vi "E5081A.vi"(5 "Input":T1={"setSweepPoint"=11, "Meas"=1, "Mark"=1, "Mark_Freq_GHz"=39.0, "Start_Freq(GHz)"=0.0, "Stop_Freq(GHz)"=0.0, "sParameter"=1}, 7 "Function_VNA":T2, 8 "error in":errorcluster, 10 "FileName":string="SENS1:CORR:CACHe:MODE 1", 11 "VISA IN":refnum<visa-resource-name>="TCPIP0::192.168.100.12::inst0::INSTR") -> (0 "error out":errorcluster, 3 "queryMarker":cluster{"gain":dbl, "phase":dbl} {"phase" format="%#.3f"; "gain" format="%#.3f"})   [LabVIEW 2023, in "Keysight.lvlib"]
uses:
  Keysight.lvlib
  CTL/Keysight_VNA.ctl
panel:
  out "Response":string
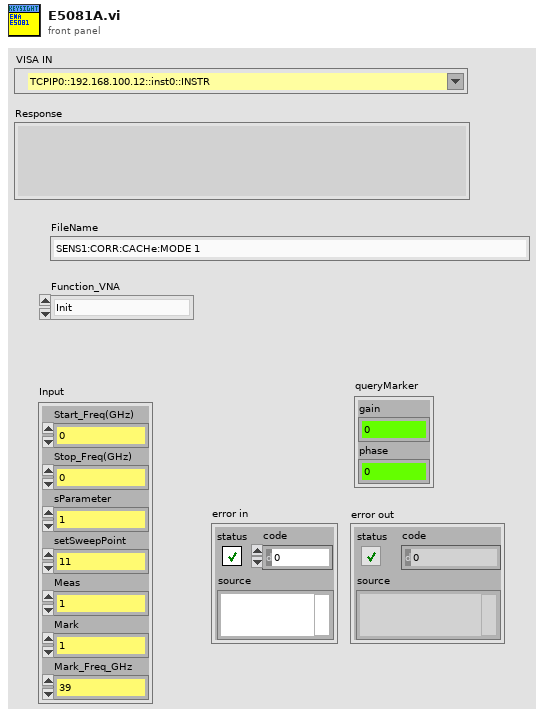
[diagram p1: front panel]
types:
  T1 = cluster{"setSweepPoint":i32, "Meas":i32, "Mark":i32, "Mark_Freq_GHz":dbl, "Start_Freq(GHz)":dbl, "Stop_Freq(GHz)":dbl, "sParameter":i32}
  T2 = typedef "Keysight_VNA.ctl" = enum16{"Init", "queryMarker", "setSweepPoint", "setMarkerFreq", "setMeasureFormat", "setFreqStartStop", "setMarkerOnOFF", "setMarkerFormat_LOGP", "setMeasPAR_S", "setTriggerSingle", "Trigger_Save_SnP", "Trigger_Single", "Close"}
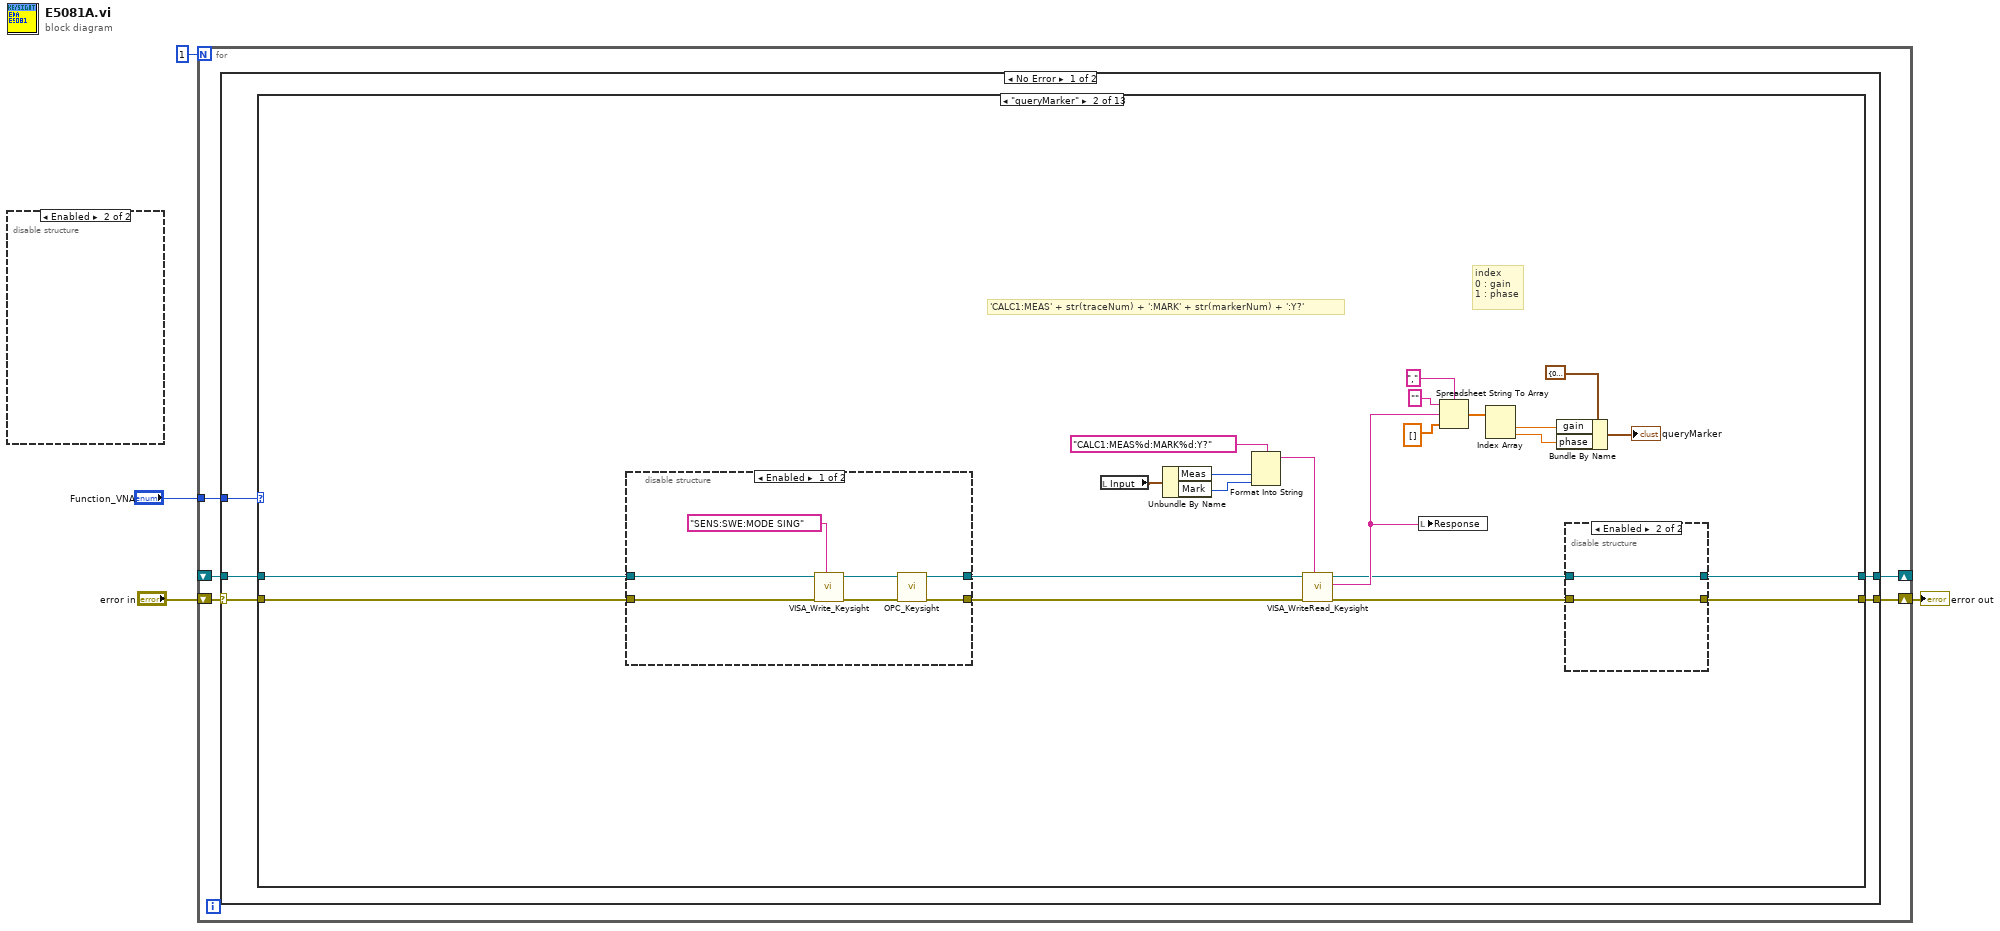
[diagram p0: block diagram]
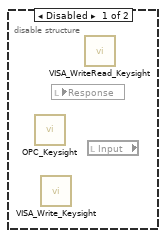
[diagram p2: hidden frame]
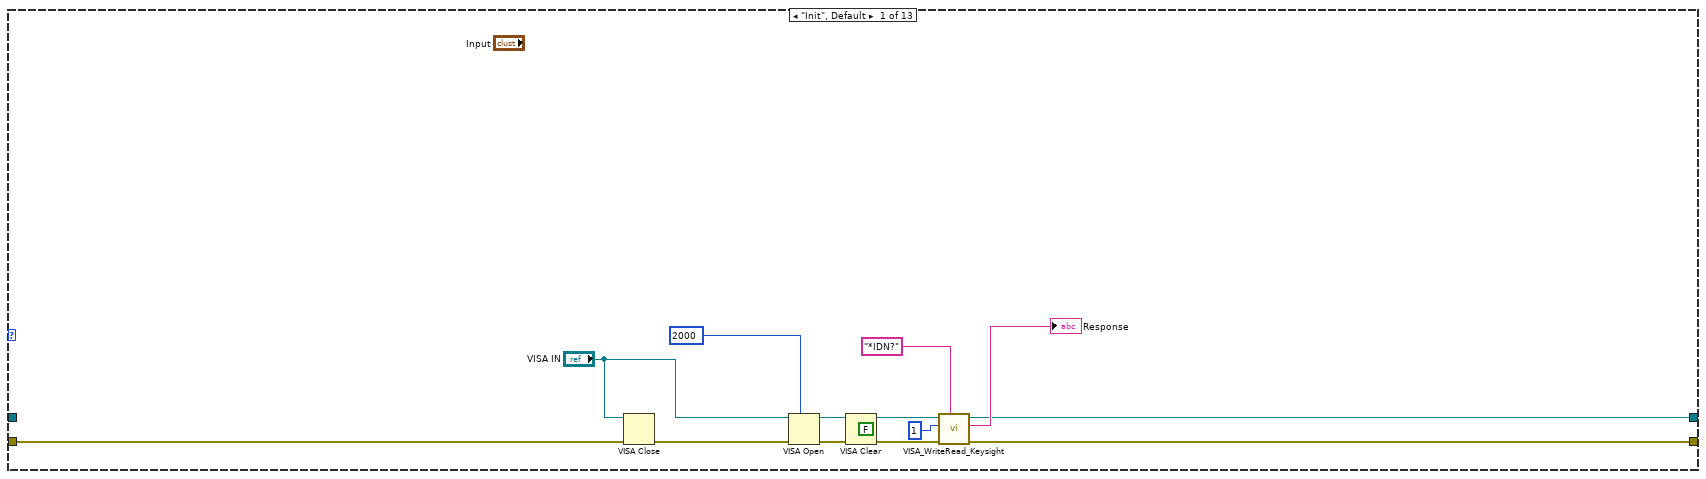
[diagram p3: hidden frame]
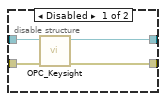
[diagram p4: hidden frame]
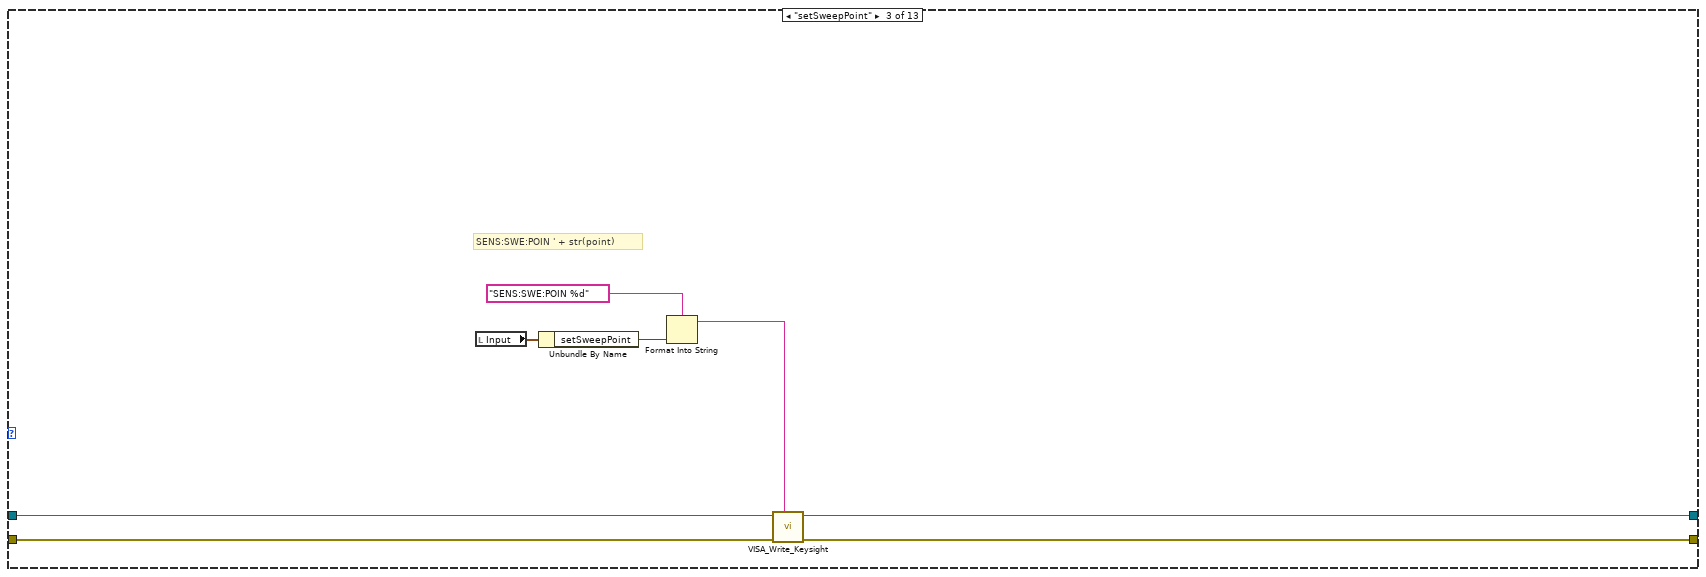
[diagram p6: hidden frame]
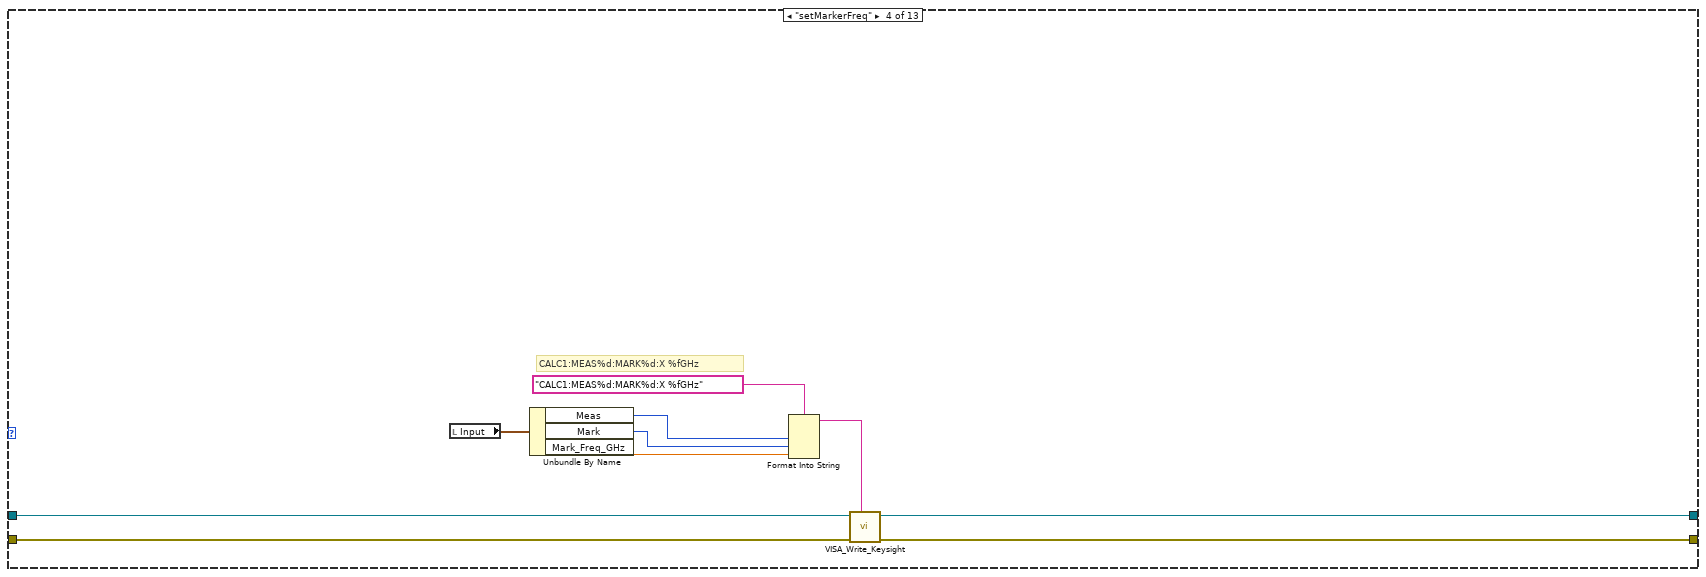
[diagram p7: hidden frame]
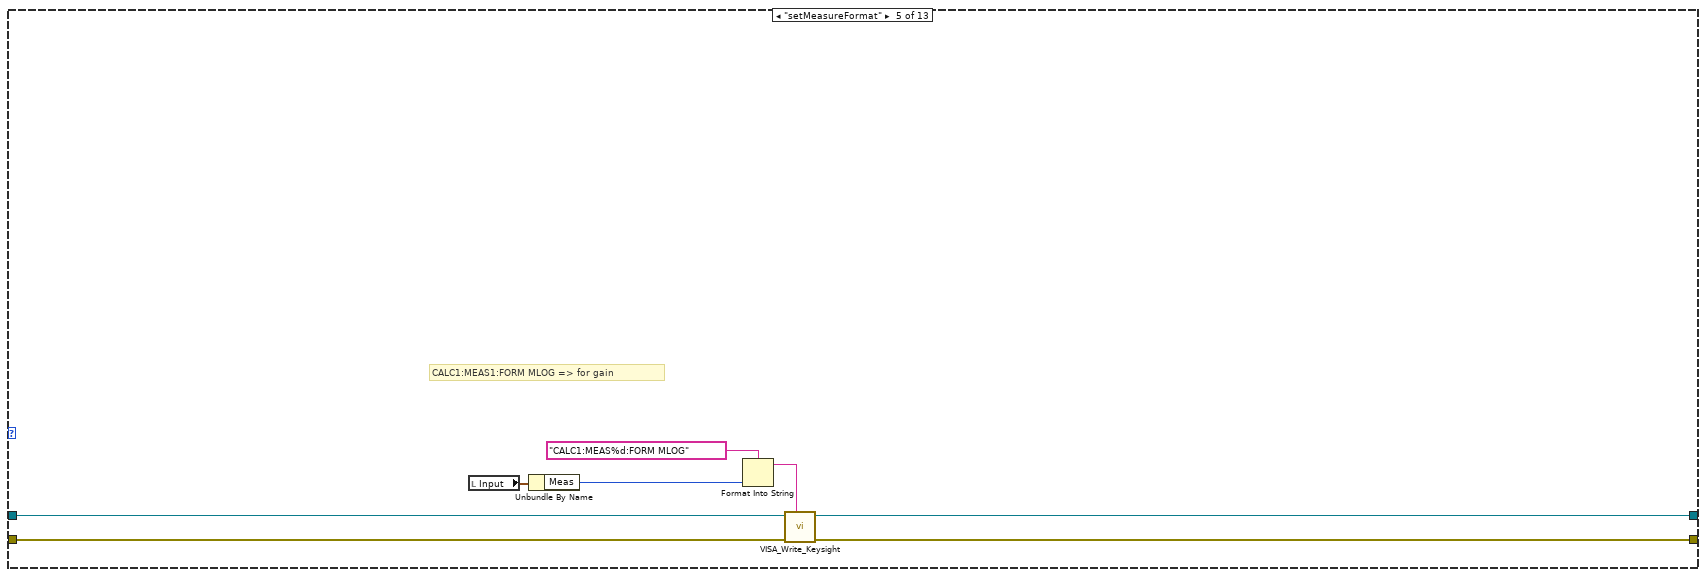
[diagram p8: hidden frame]
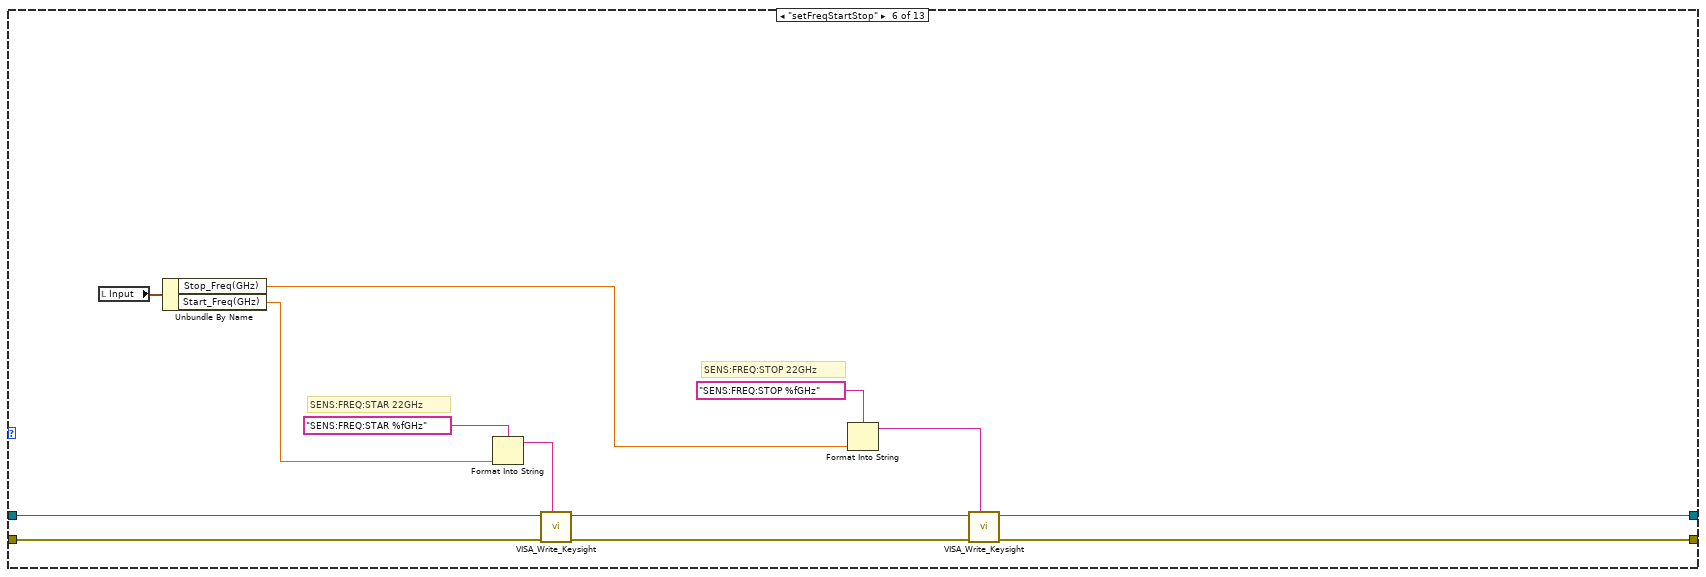
[diagram p9: hidden frame]
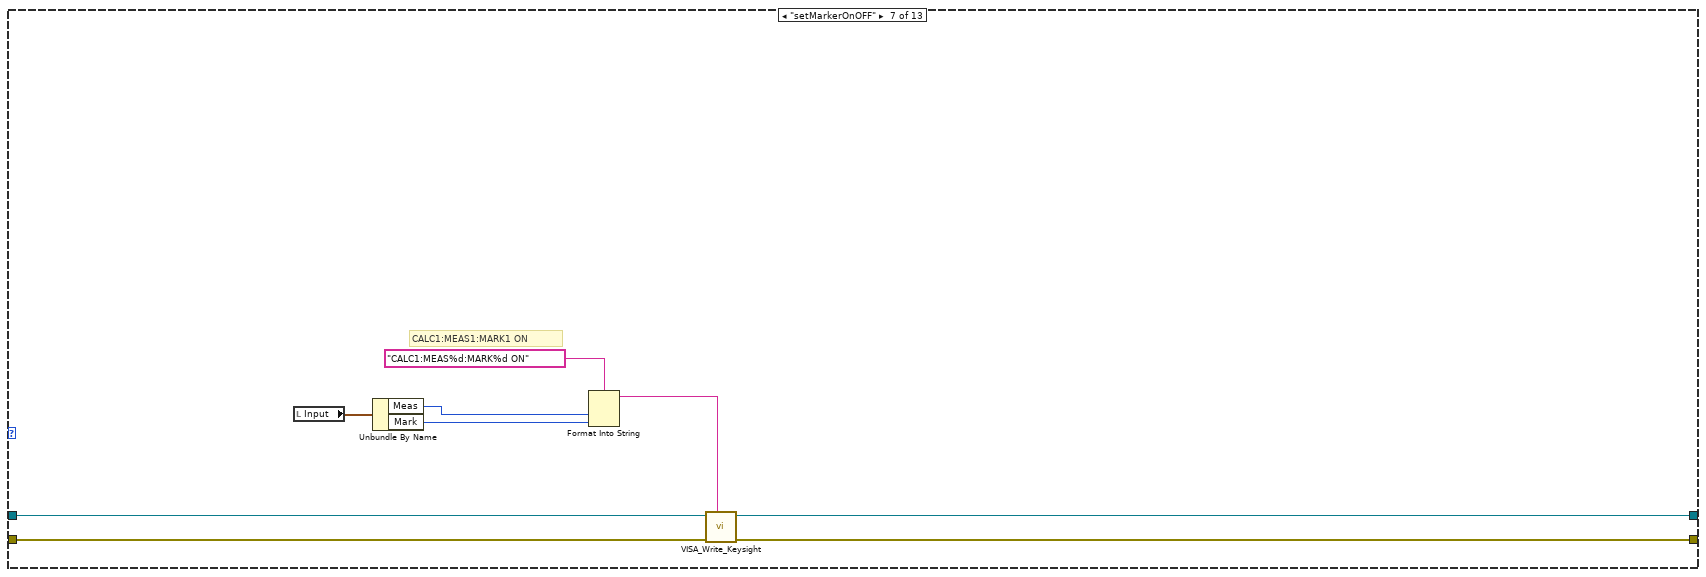
[diagram p10: hidden frame]
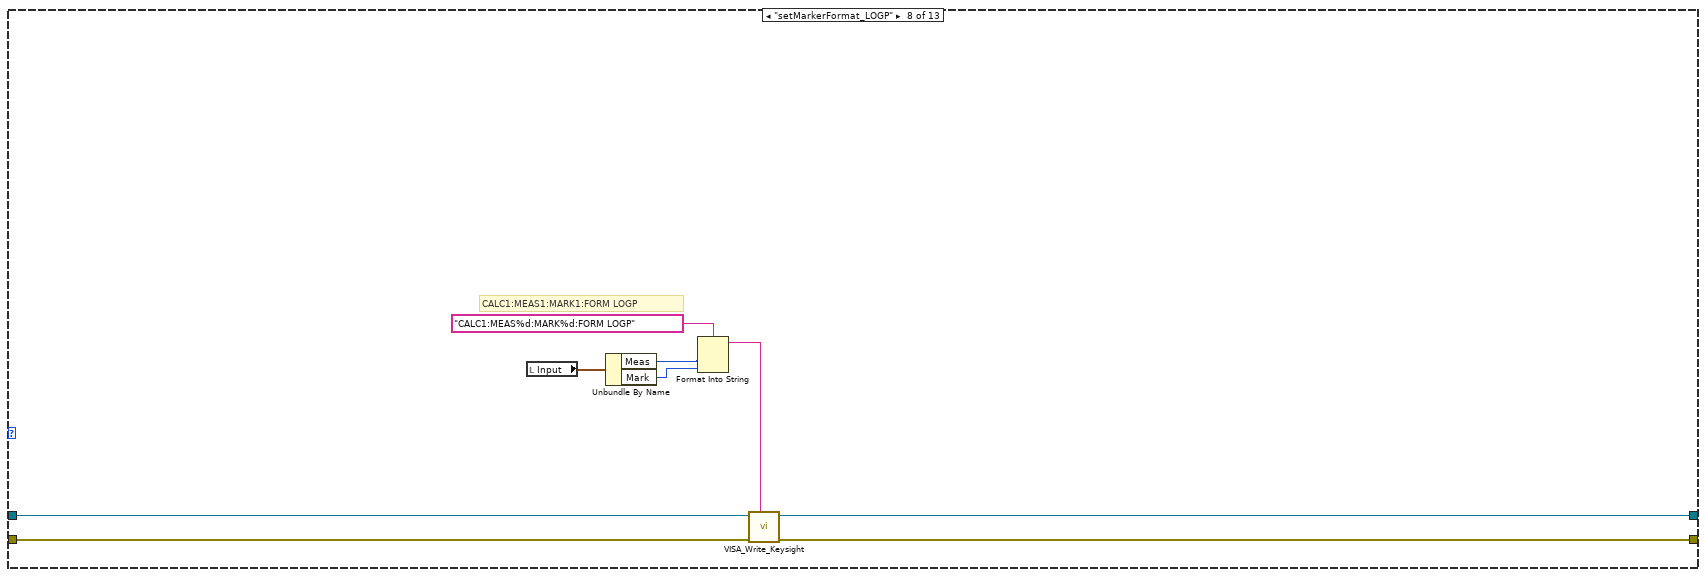
[diagram p11: hidden frame]
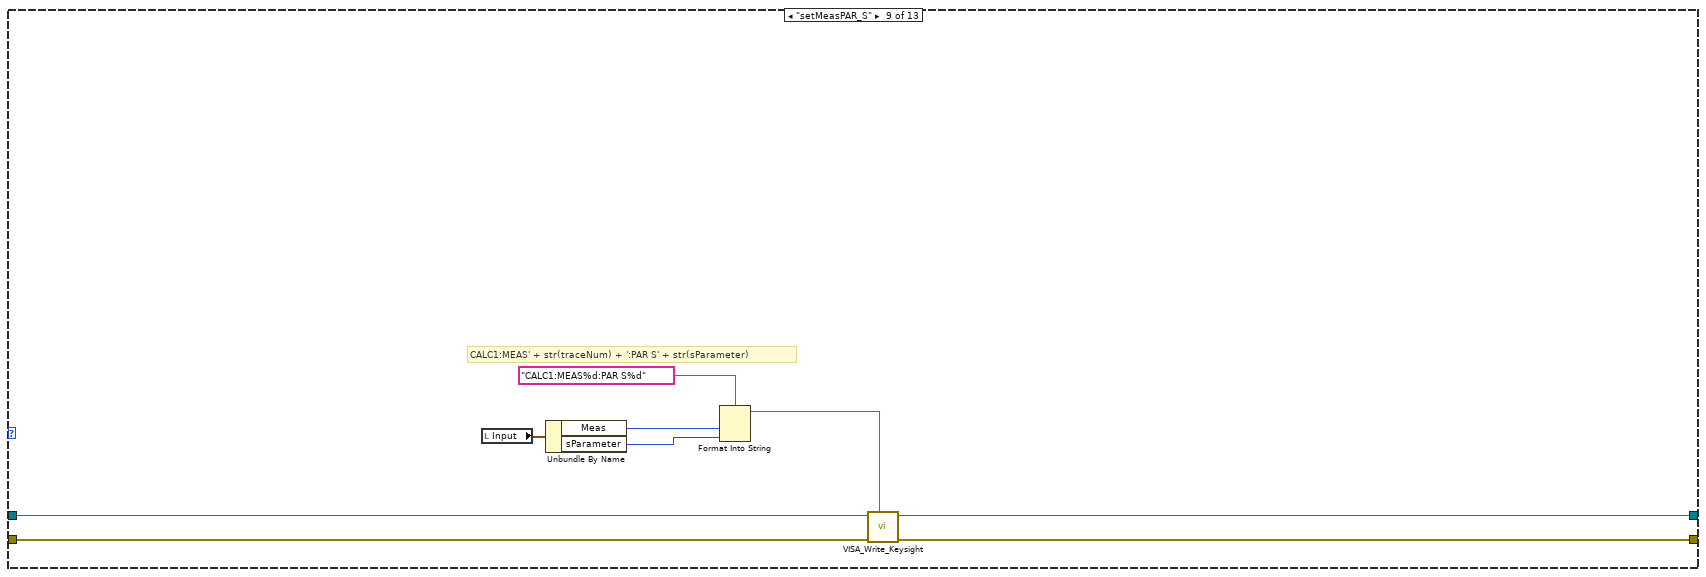
[diagram p12: hidden frame]
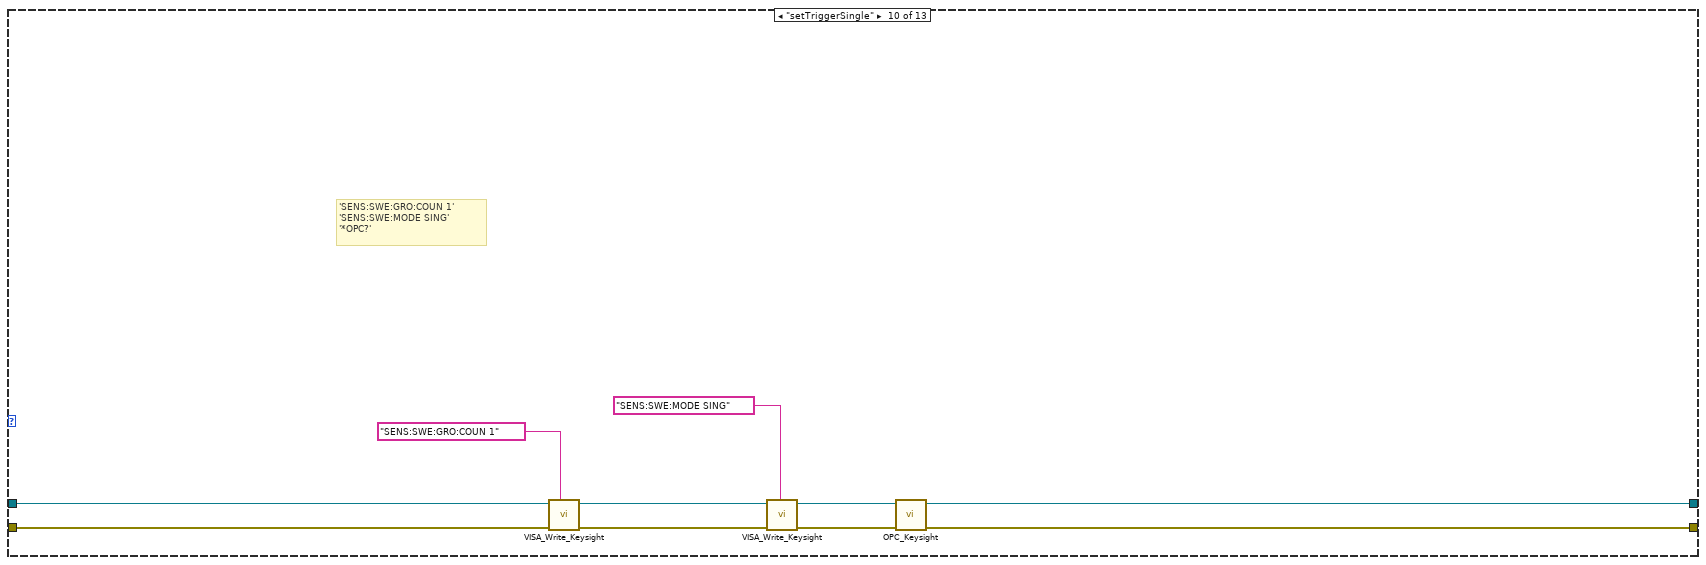
[diagram p13: hidden frame]
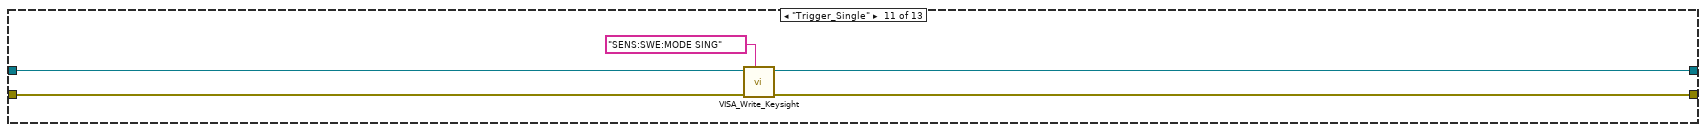
[diagram p14: hidden frame]
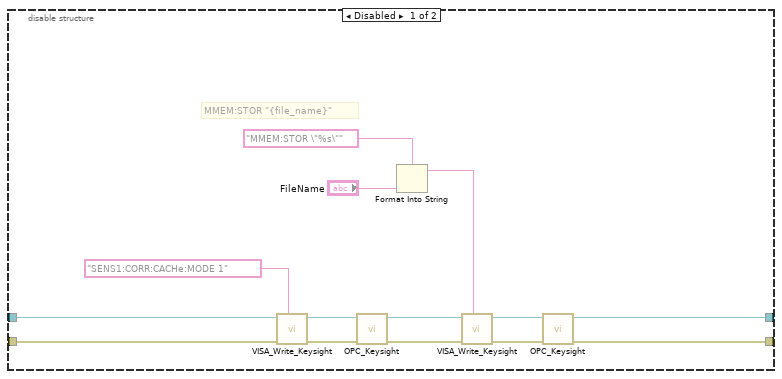
[diagram p16: hidden frame]
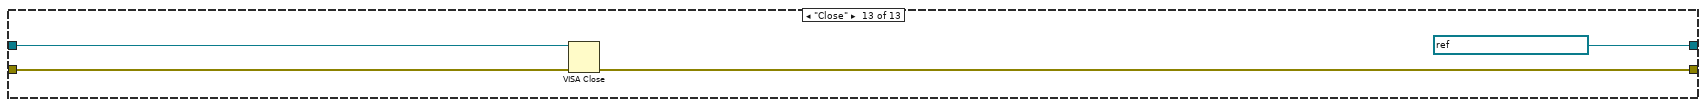
[diagram p17: hidden frame]
diagram:
  n1 = disable-structure shown="Enabled" {
    frame Disabled {
      n2 = call "OPC_Keysight.vi"() -> ()  [unwired: 10 in, 2 out]
      n3 = call "VISA_Write_Keysight.vi"() -> ()  [unwired: 10 in, 2 out]
      n4 = local read "Response"() -> ()  [unwired: 1 in]
      n5 = call "VISA_WriteRead_Keysight.vi"() -> ()  [unwired: 9 in, 3 out]
      n6 = local read "Input"() -> ()  [unwired: 1 out]
    }
    frame Enabled {
    }
  }
  n7 = for {
    N: 1 -> [_]
    tunnel: "Function_VNA" -> [w7]
    shift-right: [w8] -> w3
    shift-left: "error in" -> [w9]
    shift-right: [w5] -> _
    shift-left: _ -> [w6]
    n8 = case shown="No Error" w9 {
      selector: w9 -> [w13 w171]
      tunnel: [w11 w171] -> w8
      tunnel: w7 -> [w14 _]
      tunnel: w6 -> [w10 w170]
      tunnel: [w12 w170] -> w5
      frame No Error {
        n9 = case shown="\"queryMarker\"" w14 {
          tunnel: w13 -> [w17 w37 w70 w81 w90 w103 w112 w121 w129 w140 w144 w149 w169]
          tunnel: [w16 w34 w68 w79 w87 w95 w107 w118 w126 w134 w141 w146 refnum<visa-resource-name> refnum ("VISA out")] -> w12
          tunnel: [w15 w33 w67 w78 w89 w97 w111 w120 w128 w133 w143 w147 w167] -> w11
          tunnel: w10 -> [_ w38 w69 w80 w88 w102 w108 w119 w127 w139 w142 w148 w168]
          frame "Init", Default {
            (unwired) FALSE ("duplicate session (F)")
            n10 = VISA Close(VISA resource name="VISA IN", error in (no error)=w17) -> (error out=w24:errorcluster)
            n11 = VISA Open(timeout (0)=u32 2000 ("VISA Open timeout (0)"), error in (no error)=w24, VISA resource name="VISA IN") -> (VISA resource name=w25:refnum<visa-resource-name>, error out=w26:errorcluster)  [unwired: 2 in]
            n12 = VISA Clear(VISA resource name=w25, error in (no error)=w26) -> (VISA resource name out=w21:refnum<visa-resource-name>, error out=w22:errorcluster)
            n13 = call "VISA_WriteRead_Keysight.vi"("VISA_CMD"="*IDN?", "error in"=w22, "waiting(ms)"=u32 1, "VISA in"=w21) -> ("error out"=w15:errorcluster, "Response"=→"Response":string, "VISA out"=w16:refnum<visa-resource-name>)  [unwired: 5 in]
          }
          frame "queryMarker" {
            # "index\n0 : gain\n1 : phase"
            # "'CALC1:MEAS' + str(traceNum) + ':MARK' + str(markerNum) + ':Y?'"
            n14 = disable-structure shown="Enabled" {
              disable-tunnel: w38 -> [w62 w64]
              disable-tunnel: w37 -> [w61 w63]
              disable-tunnel: [w56 w63] -> w29
              disable-tunnel: [w57 w64] -> w28
              frame Enabled {
                n15 = call "VISA_Write_Keysight.vi"("VISA CMD"="SENS:SWE:MODE SING" ("VISA_CMD"), "error in"=w61, "VISA in"=w62) -> ("error out"=w59:errorcluster, "VISA out"=w58:refnum<visa-resource-name>)  [unwired: 7 in]
                n16 = call "OPC_Keysight.vi"("error in (no error)"=w59, "VISA resource name"=w58) -> ("error out"=w56:errorcluster, "VISA resource name out"=w57:refnum<visa-resource-name>)  [unwired: 8 in]
              }
              frame Disabled {
              }
            }
            n17 = local read "Input"() -> (w32:T1)
            n18 = Unbundle By Name(w32) -> ("Meas"=w31:i32, "Mark"=w30:i32)
            n19 = Format Into String(format string="CALC1:MEAS%d:MARK%d:Y?" ("VISA_CMD"), w31, w30) -> (resulting string=w48:string)  [unwired: 2 in, 1 out]
            n20 = call "VISA_WriteRead_Keysight.vi"("VISA_CMD"=w48, "error in"=w29, "VISA in"=w28) -> ("error out"=w36:errorcluster, "Response"=w47:string, "VISA out"=w35:refnum<visa-resource-name>)  [unwired: 6 in]
            n21 = local write "Response"(w47) -> ()
            n22 = Spreadsheet String To Array(delimiter (Tab)=",", format string="", spreadsheet string=w47, array type (2D Dbl)=dbl[] []) -> (array=w43:dbl[])
            n23 = Index Array(array=w43) -> (element #1=w41:dbl, element #2=w40:dbl)  [unwired: 2 in]
            n24 = Bundle By Name(cluster=cluster{"gain":dbl, "phase":dbl} {"gain"=0.0, "phase"=0.0} ("queryMarker 2"), "gain"=w41, "phase"=w40) -> (→"queryMarker":cluster{"gain":dbl, "phase":dbl})
            n25 = disable-structure shown="Enabled" {
              disable-tunnel: w36 -> [w53 w55]
              disable-tunnel: w35 -> [w52 w54]
              disable-tunnel: [w51 w54] -> w34
              disable-tunnel: [w50 w55] -> w33
              frame Disabled {
                n26 = call "OPC_Keysight.vi"("error in (no error)"=w53, "VISA resource name"=w52) -> ("error out"=w50:errorcluster, "VISA resource name out"=w51:refnum<visa-resource-name>)  [unwired: 8 in]
              }
              frame Enabled {
              }
            }
          }
          frame "setSweepPoint" {
            # "SENS:SWE:POIN ' + str(point)"
            n27 = local read "Input"() -> (w66:T1)
            n28 = Unbundle By Name(w66) -> ("setSweepPoint"=w65:i32)
            n29 = Format Into String(format string="SENS:SWE:POIN %d" ("write buffer"), w65) -> (resulting string=w71:string)  [unwired: 2 in, 1 out]
            n30 = call "VISA_Write_Keysight.vi"("VISA CMD"=w71, "error in"=w70, "VISA in"=w69) -> ("error out"=w67:errorcluster, "VISA out"=w68:refnum<visa-resource-name>)  [unwired: 7 in]
          }
          frame "setMarkerFreq" {
            # "CALC1:MEAS%d:MARK%d:X %fGHz"
            n31 = local read "Input"() -> (w76:T1)
            n32 = Unbundle By Name(w76) -> ("Meas"=w75:i32, "Mark"=w74:i32, "Mark_Freq_GHz"=w73:dbl)
            n33 = Format Into String(format string="CALC1:MEAS%d:MARK%d:X %fGHz" ("write buffer"), w75, w74, w73) -> (resulting string=w77:string)  [unwired: 2 in, 1 out]
            n34 = call "VISA_Write_Keysight.vi"("VISA CMD"=w77, "error in"=w81, "VISA in"=w80) -> ("error out"=w78:errorcluster, "VISA out"=w79:refnum<visa-resource-name>)  [unwired: 7 in]
          }
          frame "setMeasureFormat" {
            # "CALC1:MEAS1:FORM MLOG => for gain"
            n35 = local read "Input"() -> (w84:T1)
            n36 = Unbundle By Name(w84) -> ("Meas"=w83:i32)
            n37 = Format Into String(format string="CALC1:MEAS%d:FORM MLOG" ("VISA_CMD"), w83) -> (resulting string=w85:string)  [unwired: 2 in, 1 out]
            n38 = call "VISA_Write_Keysight.vi"("VISA CMD"=w85, "error in"=w90, "VISA in"=w88) -> ("error out"=w89:errorcluster, "VISA out"=w87:refnum<visa-resource-name>)  [unwired: 7 in]
          }
          frame "setFreqStartStop" {
            # "SENS:FREQ:STOP 22GHz"
            # "SENS:FREQ:STAR 22GHz"
            n39 = local read "Input"() -> (w93:T1)
            n40 = Unbundle By Name(w93) -> ("Stop_Freq(GHz)"=w91:dbl, "Start_Freq(GHz)"=w92:dbl)
            n41 = Format Into String(format string="SENS:FREQ:STAR %fGHz" ("write buffer"), w92) -> (resulting string=w100:string)  [unwired: 2 in, 1 out]
            n42 = call "VISA_Write_Keysight.vi"("VISA CMD"=w100, "error in"=w103, "VISA in"=w102) -> ("error out"=w98:errorcluster, "VISA out"=w96:refnum<visa-resource-name>)  [unwired: 7 in]
            n43 = Format Into String(format string="SENS:FREQ:STOP %fGHz" ("write buffer"), w91) -> (resulting string=w94:string)  [unwired: 2 in, 1 out]
            n44 = call "VISA_Write_Keysight.vi"("VISA CMD"=w94, "error in"=w98, "VISA in"=w96) -> ("error out"=w97:errorcluster, "VISA out"=w95:refnum<visa-resource-name>)  [unwired: 7 in]
          }
          frame "setMarkerOnOFF" {
            # "CALC1:MEAS1:MARK1 ON"
            n45 = local read "Input"() -> (w106:T1)
            n46 = Unbundle By Name(w106) -> ("Meas"=w105:i32, "Mark"=w104:i32)
            n47 = Format Into String(format string="CALC1:MEAS%d:MARK%d ON" ("write buffer"), w105, w104) -> (resulting string=w109:string)  [unwired: 2 in, 1 out]
            n48 = call "VISA_Write_Keysight.vi"("VISA CMD"=w109, "error in"=w112, "VISA in"=w108) -> ("error out"=w111:errorcluster, "VISA out"=w107:refnum<visa-resource-name>)  [unwired: 7 in]
          }
          frame "setMarkerFormat_LOGP" {
            # "CALC1:MEAS1:MARK1:FORM LOGP"
            n49 = local read "Input"() -> (w115:T1)
            n50 = Unbundle By Name(w115) -> ("Meas"=w114:i32, "Mark"=w113:i32)
            n51 = Format Into String(format string="CALC1:MEAS%d:MARK%d:FORM LOGP" ("write buffer"), w114, w113) -> (resulting string=w116:string)  [unwired: 2 in, 1 out]
            n52 = call "VISA_Write_Keysight.vi"("VISA CMD"=w116, "error in"=w121, "VISA in"=w119) -> ("error out"=w120:errorcluster, "VISA out"=w118:refnum<visa-resource-name>)  [unwired: 7 in]
          }
          frame "setMeasPAR_S" {
            # "CALC1:MEAS' + str(traceNum) + ':PAR S' + str(sParameter)"
            n53 = local read "Input"() -> (w124:T1)
            n54 = Unbundle By Name(w124) -> ("Meas"=w123:i32, "sParameter"=w122:i32)
            n55 = Format Into String(format string="CALC1:MEAS%d:PAR S%d" ("write buffer"), w123, w122) -> (resulting string=w125:string)  [unwired: 2 in, 1 out]
            n56 = call "VISA_Write_Keysight.vi"("VISA CMD"=w125, "error in"=w129, "VISA in"=w127) -> ("error out"=w128:errorcluster, "VISA out"=w126:refnum<visa-resource-name>)  [unwired: 7 in]
          }
          frame "setTriggerSingle" {
            # "'SENS:SWE:GRO:COUN 1'\n'SENS:SWE:MODE SING'\n'*OPC?'"
            n57 = call "VISA_Write_Keysight.vi"("VISA CMD"="SENS:SWE:GRO:COUN 1" ("write buffer"), "error in"=w140, "VISA in"=w139) -> ("error out"=w138:errorcluster, "VISA out"=w137:refnum<visa-resource-name>)  [unwired: 7 in]
            n58 = call "VISA_Write_Keysight.vi"("VISA CMD"="SENS:SWE:MODE SING" ("write buffer"), "error in"=w138, "VISA in"=w137) -> ("error out"=w135:errorcluster, "VISA out"=w136:refnum<visa-resource-name>)  [unwired: 7 in]
            n59 = call "OPC_Keysight.vi"("error in (no error)"=w135, "VISA resource name"=w136) -> ("error out"=w133:errorcluster, "VISA resource name out"=w134:refnum<visa-resource-name>)  [unwired: 8 in]
          }
          frame "Trigger_Single" {
            n60 = call "VISA_Write_Keysight.vi"("VISA CMD"="SENS:SWE:MODE SING" ("write buffer"), "error in"=w144, "VISA in"=w142) -> ("error out"=w143:errorcluster, "VISA out"=w141:refnum<visa-resource-name>)  [unwired: 7 in]
          }
          frame "Trigger_Save_SnP" {
            n61 = disable-structure shown="Enabled" {
              disable-tunnel: w149 -> [w163 w165]
              disable-tunnel: w148 -> [w162 w164]
              disable-tunnel: [w151 w165] -> w147
              disable-tunnel: [w150 w164] -> w146
              frame Disabled {
                # "MMEM:STOR \"{file_name}\""
                n62 = call "VISA_Write_Keysight.vi"("VISA CMD"="SENS1:CORR:CACHe:MODE 1" ("write buffer"), "error in"=w163, "VISA in"=w162) -> ("error out"=w161:errorcluster, "VISA out"=w160:refnum<visa-resource-name>)  [unwired: 7 in]
                n63 = call "OPC_Keysight.vi"("error in (no error)"=w161, "VISA resource name"=w160) -> ("error out"=w159:errorcluster, "VISA resource name out"=w158:refnum<visa-resource-name>)  [unwired: 8 in]
                n64 = Format Into String(format string="MMEM:STOR \"%s\"" ("write buffer"), "FileName") -> (resulting string=w152:string)  [unwired: 2 in, 1 out]
                n65 = call "VISA_Write_Keysight.vi"("VISA CMD"=w152, "error in"=w159, "VISA in"=w158) -> ("error out"=w157:errorcluster, "VISA out"=w156:refnum<visa-resource-name>)  [unwired: 7 in]
                n66 = call "OPC_Keysight.vi"("error in (no error)"=w157, "VISA resource name"=w156) -> ("error out"=w151:errorcluster, "VISA resource name out"=w150:refnum<visa-resource-name>)  [unwired: 8 in]
              }
              frame Enabled {
              }
            }
          }
          frame "Close" {
            n67 = VISA Close(VISA resource name=w168, error in (no error)=w169) -> (error out=w167:errorcluster)
          }
        }
      }
      frame Error {
      }
    }
  }
  "error out" <- w3
